vi "Stop Log.vi"(8 "error in (no error)":errorcluster, 11 "Data Logger Module in":refnum<class "Data Logger DBL Module.lvclass">) -> (0 "error out":errorcluster, 3 "Data Logger Module out":refnum<class "Data Logger DBL Module.lvclass">)   [LabVIEW 2020, in "VolatusData.lvlib" / "Data Logger DBL Module.lvclass"]
uses:
  Data Logger DBL Module.lvclass
  C:/dev/lv20CE/relink/lv-volatus/Volatus/Module/Module.lvclass
  Data Logger DBL Module.lvclass/Data Logger DBL Module.ctl
  Logger Stopped.ctl
  Logger State.ctl
  Volatus/Module/Module.lvclass/Module.ctl
  Volatus/MessageQ/MessageQ.lvclass/MessageQ.ctl
  Volatus/Module/Parent Q.vi
  Volatus/Module/Update Substatus.vi
  Volatus/MessageQ/MessageQ.lvclass
  VolatusData.lvlib
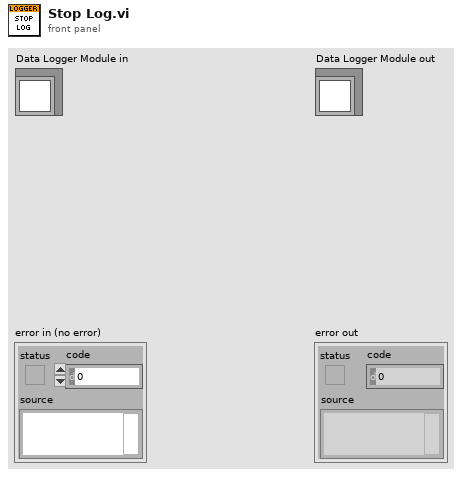
[diagram p1: front panel]
types:
  T1 = typedef "VolatusData.lvlib/Logger State.ctl" = enum16{"Unknown", "Idle", "Preparing", "Ready", "Logging", "Stopping"}
  T2 = typedef "VolatusData.lvlib/Logger Stopped.ctl" = cluster{"ID":string}
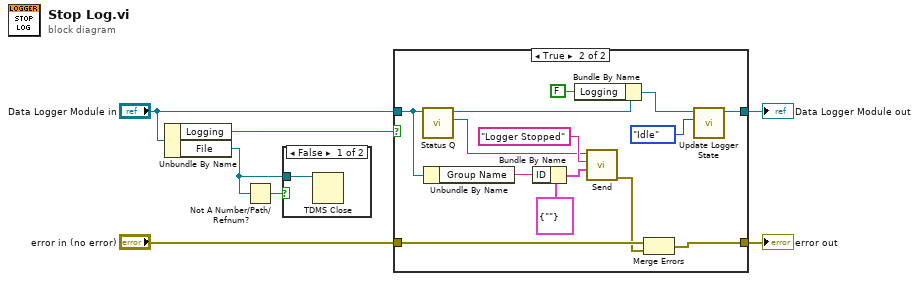
[diagram p0: block diagram]
diagram:
  n1 = Unbundle By Name("Data Logger Module in") -> ("Logging"=w5:bool, "File"=w6:refnum<k34>)
  n2 = Not A Number/Path/Refnum?(number/path/refnum=w6) -> (NaN/Path/Refnum?=w7:bool)
  n3 = case shown="False" w7 {
    tunnel: w6 -> [w8 _]
    frame False {
      n4 = TDMS Close(11:w8) -> ()  [unwired: 1 in, 2 out]
    }
    frame True {
    }
  }
  n5 = case shown="True" w5 {
    tunnel: "error in (no error)" -> [w10 w21]
    tunnel: "Data Logger Module in" -> [w9 w12]
    tunnel: [w10 w19] -> w2
    tunnel: [w9 w16] -> w1
    frame False {
    }
    frame True {
      n6 = call "Status Q.vi"("Data Logger Module in"=w12) -> ("Status Q"=w13:refnum<class "MessageQ.lvclass">, "Data Logger Module out"=w14:refnum<class "Data Logger DBL Module.lvclass">)  [unwired: 9 in]
      n7 = Unbundle By Name(w12) -> ("Group Name"=w11:string)
      n8 = Bundle By Name(cluster=T2 {"ID"=""} ("Logger Stopped"), "ID"=w11) -> (w23:T2)
      n9 = Bundle By Name(cluster=w14, "Logging"=FALSE) -> (w17:refnum<class "Data Logger DBL Module.lvclass">)
      n10 = call "Send.vi"("Data"=w23, "ID"="Logger Stopped", "MessageQ in"=w13) -> ("error out"=w20:errorcluster)  [unwired: 7 in, 1 out]
      n11 = Merge Errors(w21, w20) -> (w19:errorcluster)
      n12 = call "Update Logger State.vi"("Logger State"=Logger_State."Idle", "Module in"=w17) -> ("Module"=w16:refnum<class "Data Logger DBL Module.lvclass">)  [unwired: 8 in, 1 out]
    }
  }
  "error out" <- w2
  "Data Logger Module out" <- w1
